vi "Set Switch.vi"(7 "ON/OFF":bool, 8 "error in (no error)":errorcluster, 10 "Pin":u16, 11 "PEU in":refnum<class "PEU.lvclass">) -> (0 "error out":errorcluster, 3 "PEU out":refnum<class "PEU.lvclass">)   [LabVIEW 2020, in "PEU.lvlib" / "PEU.lvclass"]
uses:
  PEU.lvclass
  PEU.lvclass/PEU.ctl
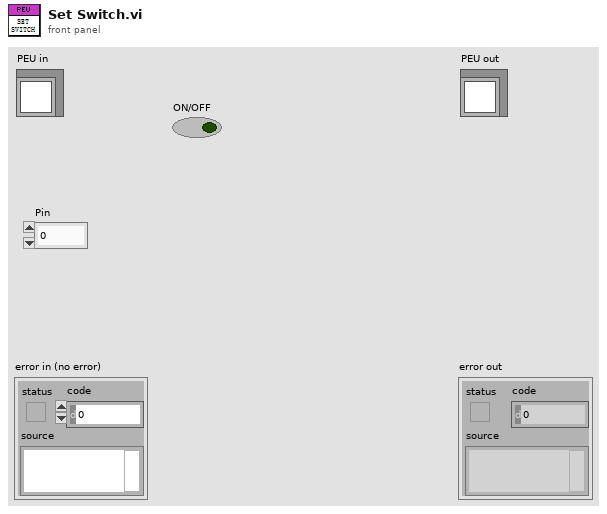
[diagram p1: front panel]
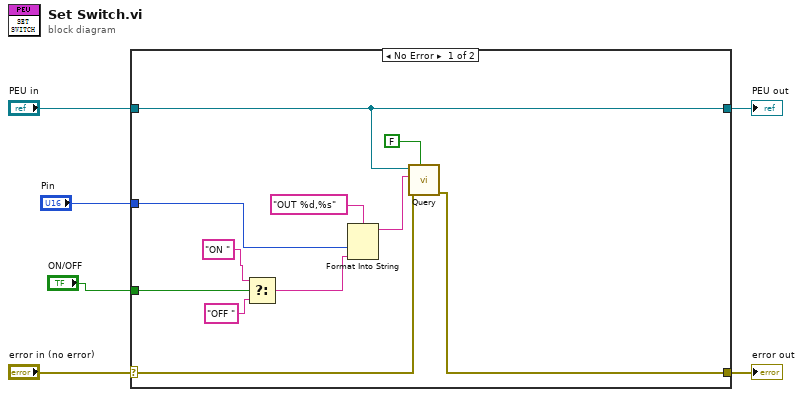
[diagram p0: block diagram]
diagram:
  n1 = case shown="No Error" "error in (no error)" {
    selector: "error in (no error)" -> [w9 w19]
    tunnel: [w7 w19] -> w5
    tunnel: [w17 w18] -> w3
    tunnel: "PEU in" -> [w17 w18]
    tunnel: "Pin" -> [w12 _]
    tunnel: "ON/OFF" -> [w8 _]
    frame No Error {
      n2 = Select(t="ON ", s=w8, f="OFF ") -> (s? t:f=w11:string)
      n3 = Format Into String(format string="OUT %d,%s", w12, w11) -> (resulting string=w10:string)  [unwired: 2 in, 1 out]
      n4 = call "Query.vi"("Return"=FALSE, "error in (no error)"=w9, "Command"=w10, "PEU in"=w17) -> ("error out"=w7:errorcluster)  [unwired: 5 in, 2 out]
    }
    frame Error {
    }
  }
  "error out" <- w5
  "PEU out" <- w3
